vi "c_ctre_phoenix6_platform_replay_is_file_loaded.vi"(0 "Numeric":u8) -> ()   [LabVIEW 2023]
uses:
  <vilib>/Rock Robotics/WPI/ThirdParty/Phoenix-LabVIEW/Controls/DriverLib.ctl
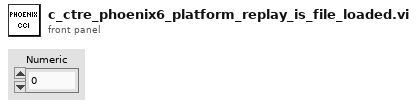
[diagram p1: front panel]
types:
  T1 = typedef "DriverLib.ctl" = path
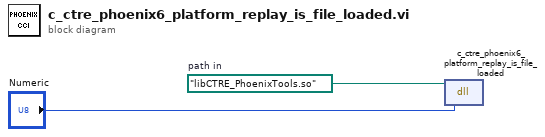
[diagram p0: block diagram]
diagram:
  w2 = T1 path "libCTRE_PhoenixTools.so"  # path in
  n1 = dll-call lib="?" fn="c_ctre_phoenix6_platform_replay_is_file_loaded"(path in=w2, "Numeric") -> ()  [unwired: 2 in, 2 out]
